vi "bigcryo-H-read.vi"(10 "Pause off":bool, 11 "Magnet Power supply":refnum<visa-resource-name>="COM6") -> (1 "substring":string="0", 3 "Magnetic Field [T]":dbl)   [LabVIEW 2019]
panel:
  out "error out":errorcluster={"status"=TRUE, "code"=-1073807339, "source"="VISA Read in bigcryo-H-read.vi"}
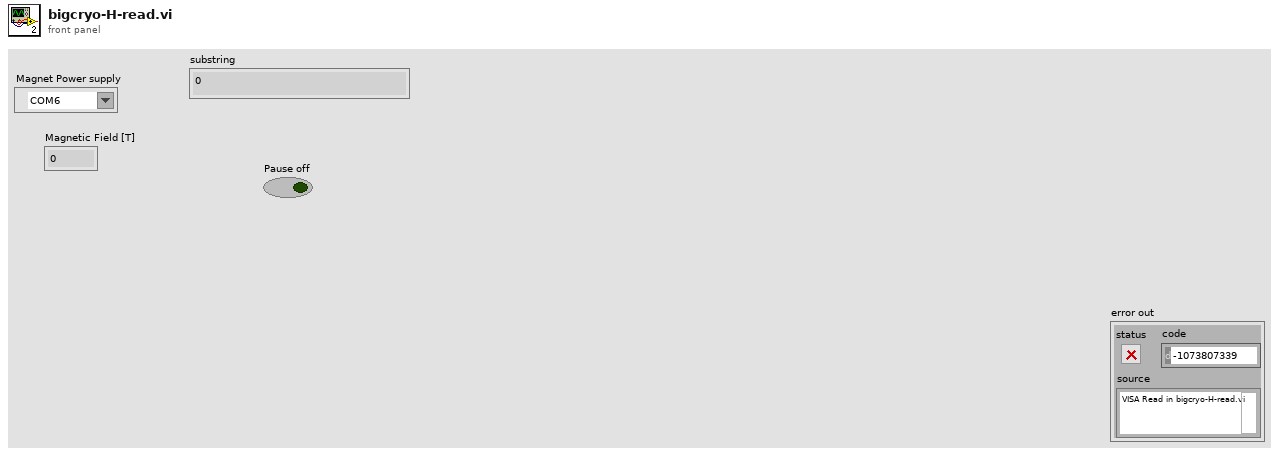
[diagram p1: front panel]
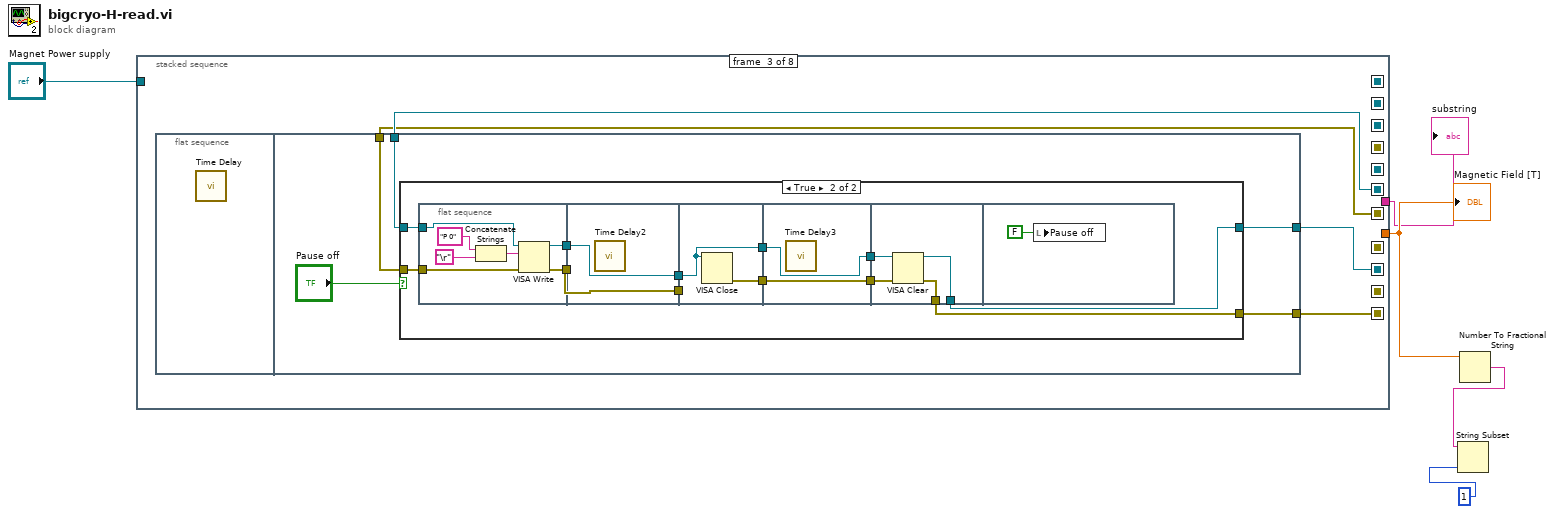
[diagram p0: block diagram]
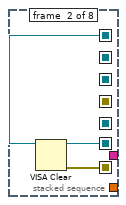
[diagram p3: hidden frame]
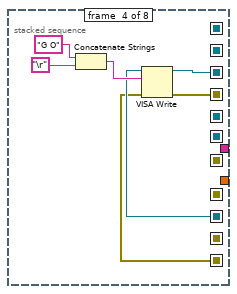
[diagram p5: hidden frame]
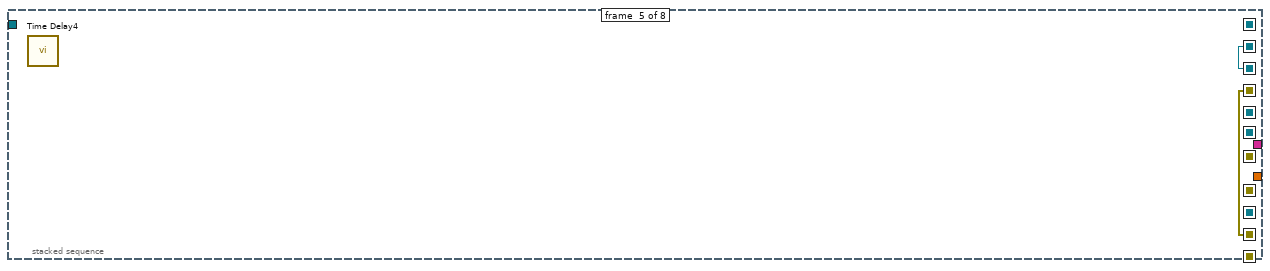
[diagram p6: hidden frame]
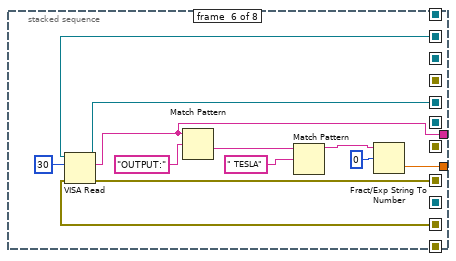
[diagram p7: hidden frame]
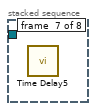
[diagram p8: hidden frame]
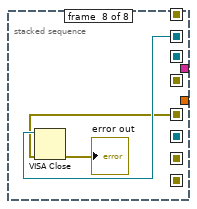
[diagram p9: hidden frame]
diagram:
  n1 = stacked-sequence {
    seq-local: [w6 _ _ _ _ _ _ _] -> [_ w9 _ _ _ _ _ _]
    seq-local: [_ w7 _ _ _ _ _ _] -> [_ _ w13 _ _ _ _ _]
    seq-local: [_ w8 _ _ _ _ _ _] -> [_ _ w10 _ _ _ _ _]
    seq-local: [_ _ w12 _ _ _ _ _] -> [_ _ _ w53 _ _ _ _]
    seq-local: [_ _ w11 _ _ _ _ _] -> [_ _ _ w52 _ _ _ _]
    seq-local: [_ _ _ w55 _ _ _ _] -> [_ _ _ _ w58 _ _ _]
    seq-local: [_ _ _ w54 _ _ _ _] -> [_ _ _ _ w59 _ _ _]
    seq-local: [_ _ _ _ w58 _ _ _] -> [_ _ _ _ _ w70 _ _]
    seq-local: [_ _ _ _ w59 _ _ _] -> [_ _ _ _ _ w68 _ _]
    seq-local: [_ _ _ _ _ w69 _ _] -> [_ _ _ _ _ _ _ w74]
    seq-local: [_ _ _ _ _ w67 _ _] -> [_ _ _ _ _ _ _ w73]
    tunnel: "Magnet Power supply" -> [w6 _ _ _ _ _ _ _]
    tunnel: [_ _ _ _ _ w61 _ _] -> w4
    tunnel: [_ _ _ _ _ w60 _ _] -> w1
    frame #0 {
    }
    frame #1 {
      n2 = VISA Clear(VISA resource name=w9) -> (VISA resource name out=w7:refnum<visa-resource-name>, error out=w8:errorcluster)  [unwired: 1 in]
    }
    frame #2 {
      n3 = flat-sequence {
        tunnel: w13 -> [w17]
        tunnel: [w16] -> w12
        tunnel: [w15] -> w11
        tunnel: w10 -> [w14]
        frame #0 {
          n4 = call "Time Delay"() -> ()  [unwired: 11 in, 1 out]
        }
        frame #1 {
          n5 = case shown="True" "Pause off" {
            tunnel: w17 -> [w20 w32]
            tunnel: [w20 w21] -> w16
            tunnel: [w19 w24] -> w15
            tunnel: w14 -> [w19 w27]
            frame False {
            }
            frame True {
              n6 = flat-sequence {
                tunnel: w32 -> [w36]
                tunnel: [w35] -> w30
                tunnel: [w34] -> w28
                tunnel: w27 -> [w33]
                tunnel: [w41] -> w31
                tunnel: w30 -> [w41]
                tunnel: [w40] -> w29
                tunnel: w28 -> [w40]
                tunnel: w31 -> [w43]
                tunnel: w29 -> [_]
                tunnel: [w43] -> w26
                tunnel: [w42] -> w22
                tunnel: w26 -> [w45]
                tunnel: [w45] -> w25
                tunnel: [w44] -> w23
                tunnel: w22 -> [w44]
                tunnel: [w49] -> w21
                tunnel: w25 -> [w48]
                tunnel: [w47] -> w24
                tunnel: w23 -> [w46]
                frame #0 {
                  n7 = Concatenate Strings("P 0" ("Command"), "\r") -> (w38:string)
                  n8 = VISA Write(VISA resource name=w36, write buffer=w38, error in (no error)=w33) -> (VISA resource name out=w35:refnum<visa-resource-name>, error out=w34:errorcluster)  [unwired: 1 out]
                }
                frame #1 {
                  n9 = call "Time Delay2"() -> ()  [unwired: 11 in, 1 out]
                }
                frame #2 {
                  n10 = VISA Close(VISA resource name=w43) -> (error out=w42:errorcluster)  [unwired: 1 in]
                }
                frame #3 {
                  n11 = call "Time Delay3"() -> ()  [unwired: 11 in, 1 out]
                }
                frame #4 {
                  n12 = VISA Clear(VISA resource name=w48, error in (no error)=w46) -> (VISA resource name out=w49:refnum<visa-resource-name>, error out=w47:errorcluster)
                }
                frame #5 {
                  n13 = local write "Pause off"(FALSE) -> ()
                }
              }
            }
          }
        }
      }
    }
    frame #3 {
      n14 = Concatenate Strings("G O" ("Command"), "\r") -> (w56:string)
      n15 = VISA Write(VISA resource name=w53, write buffer=w56, error in (no error)=w52) -> (VISA resource name out=w55:refnum<visa-resource-name>, error out=w54:errorcluster)  [unwired: 1 out]
    }
    frame #4 {
      n16 = call "Time Delay4"() -> ()  [unwired: 11 in, 1 out]
    }
    frame #5 {
      n17 = VISA Read(VISA resource name=w70, byte count=u32 30, error in (no error)=w68) -> (VISA resource name out=w69:refnum<visa-resource-name>, read buffer=w60:string, error out=w67:errorcluster)  [unwired: 1 out]
      n18 = Match Pattern(string=w60, regular expression="OUTPUT:") -> (after substring=w63:string)  [unwired: 1 in, 3 out]
      n19 = Match Pattern(string=w63, regular expression=" TESLA") -> (before substring=w62:string)  [unwired: 1 in, 3 out]
      n20 = Fract/Exp String To Number(string=w62, offset=0) -> (number=w61:dbl)  [unwired: 2 in, 1 out]
    }
    frame #6 {
      n21 = call "Time Delay5"() -> ()  [unwired: 11 in, 1 out]
    }
    frame #7 {
      n22 = VISA Close(VISA resource name=w74, error in (no error)=w73) -> (error out=→"error out":errorcluster)
    }
  }
  "Magnetic Field [T]" <- w4
  "substring" <- w1
  n23 = Number To Fractional String(number=w4) -> (F-format string=w2:string)  [unwired: 3 in]
  n24 = String Subset(string=w2, length (rest)=1 ("length (rest)")) -> ()  [unwired: 1 in, 1 out]
